vi "process_number.vi"(11 "expression":string) -> (1 "position":u16, 2 "value":dbl)   [LabVIEW 2021]
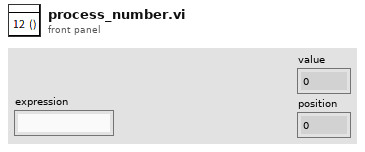
[diagram p1: front panel]
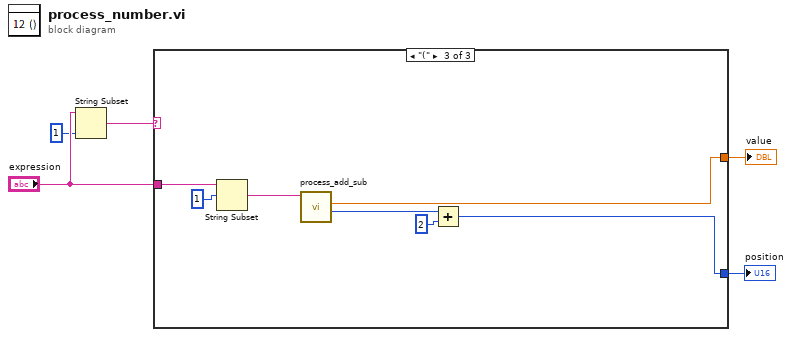
[diagram p0: block diagram]
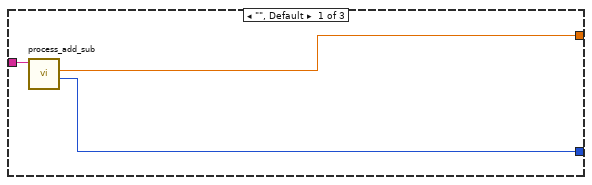
[diagram p2: hidden frame]
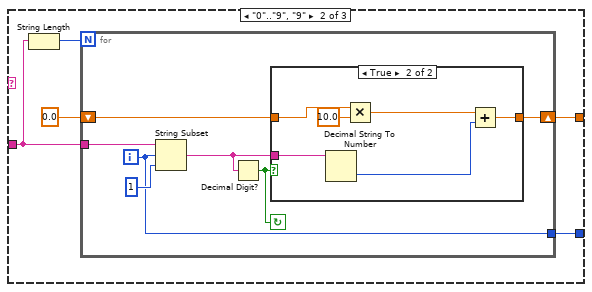
[diagram p3: hidden frame]
diagram:
  n1 = String Subset(string="expression", length (rest)=1 ("length (rest)")) -> (substring=w5:string)  [unwired: 1 in]
  n2 = case shown="\"(\"" w5 {
    tunnel: "expression" -> [w8 w10 w33]
    tunnel: [w7 w12 w34] -> w4
    tunnel: [w6 w11 w29] -> w3
    frame "", Default {
      n3 = call "process_add_sub.vi"("expression"=w8) -> ("position"=w6:u16, "value"=w7:dbl)  [unwired: 8 in]
    }
    frame "0".."9", "9" {
      n4 = String Length(string=w10) -> (length=w9:i32)
      n5 = for {
        N: w9 -> [_]
        tunnel: w10 -> [w16]
        tunnel: [w15] -> w11
        shift-right: [w19] -> w12
        shift-left: 0.0 -> [w18]
        i -> [w15]
        stop <- w20 continue-if-true
        n6 = String Subset(string=w16, offset (0)=w15, length (rest)=1 ("length (rest)")) -> (substring=w14:string)
        n7 = Decimal Digit?(1:w14) -> (0:w20:bool)
        n8 = case shown="True" w20 {
          tunnel: w14 -> [_ w27]
          tunnel: [w21 w23] -> w19
          tunnel: w18 -> [w21 w22]
          frame False {
          }
          frame True {
            n9 = Decimal String To Number(string=w27) -> (number=w24:i32)  [unwired: 2 in, 1 out]
            n10 = Multiply(x=w22, y=10.0) -> (x*y=w26:dbl)
            n11 = Add(x=w26, y=w24) -> (x+y=w23:dbl)
          }
        }
      }
    }
    frame "(" {
      n12 = String Subset(string=w33, offset (0)=1 ("index")) -> (substring=w32:string)  [unwired: 1 in]
      n13 = call "process_add_sub.vi"("expression"=w32) -> ("position"=w31:u16, "value"=w34:dbl)  [unwired: 8 in]
      n14 = Add(x=w31, y=u16 2) -> (x+y=w29:u16)
    }
  }
  "value" <- w4
  "position" <- w3
